vi "Query Slewrate Limits.vi"(7 "Channel (0: Channel A)":u16(ring) items=["Channel A", "Channel B"], 8 "error in (no error)":errorcluster, 11 "BH Druck PACE Series in":refnum<class "BH Druck PACE Series.lvclass">) -> (0 "error out":errorcluster, 1 "Lower Slew Rate Limit":dbl, 2 "Upper Slew Rate Limit":dbl, 3 "BH Druck PACE Series out":refnum<class "BH Druck PACE Series.lvclass">)   [LabVIEW 2022 SP3, in "BH Druck PACE Series.lvclass"]
uses:
  BH Druck PACE Series.lvclass
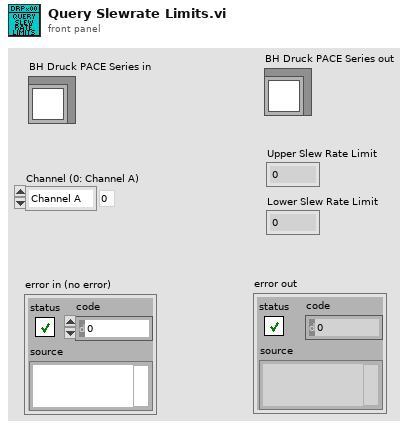
[diagram p1: front panel]
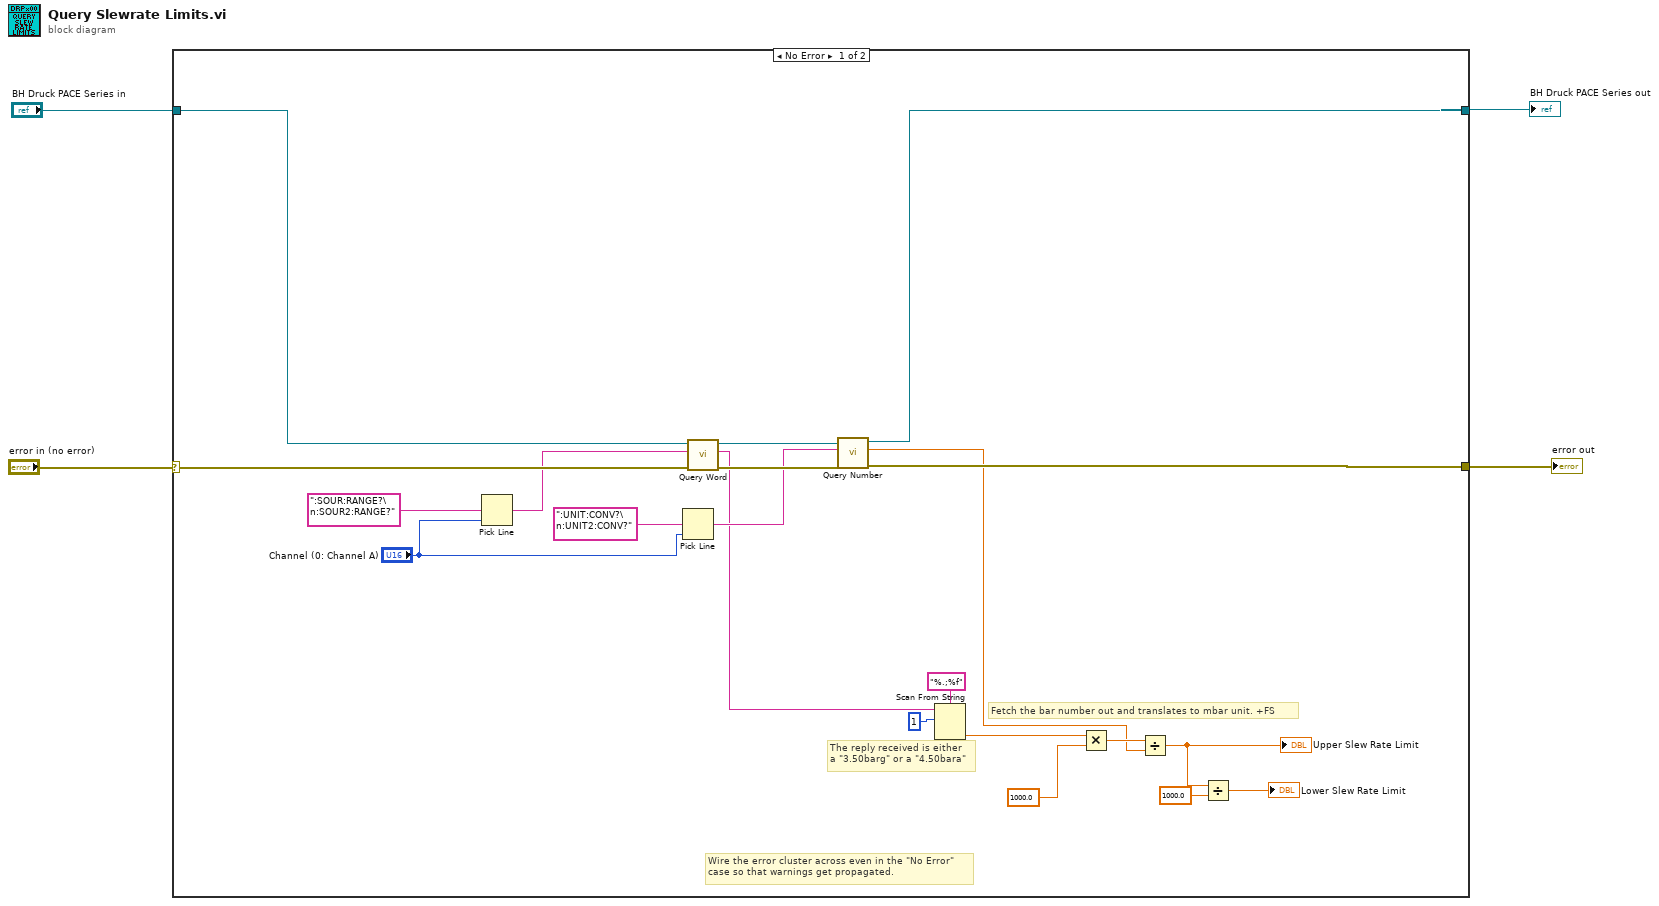
[diagram p0: block diagram]
diagram:
  n1 = case shown="No Error" "error in (no error)" {
    selector: "error in (no error)" -> [w22 w27]
    tunnel: [w20 w27] -> w3
    tunnel: [w16 w26] -> w1
    tunnel: "BH Druck PACE Series in" -> [w19 w26]
    frame No Error {
      # "Fetch the bar number out and translates to mbar unit. +FS"
      # "The reply received is either \na \"3.50barg\" or a \"4.50bara\""
      # "Wire the error cluster across even in the \"No Error\"\ncase so that warnings get propagated."
      n2 = Pick Line(multi-line string=":SOUR:RANGE?\n:SOUR2:RANGE?", line index="Channel (0: Channel A)") -> (output string=w15:string)  [unwired: 1 in]
      n3 = Pick Line(multi-line string=":UNIT:CONV?\n:UNIT2:CONV?", line index="Channel (0: Channel A)") -> (output string=w17:string)  [unwired: 1 in]
      n4 = call-dynamic "Query Word.vi"("error in (no error)"=w22, "Query String"=w15, "BH Druck PACE Series in"=w19) -> ("error out"=w21:errorcluster, "String Result"=w6:string, "BH Druck PACE Series out"=w18:refnum<class "BH Druck PACE Series.lvclass">)  [unwired: 6 in]
      n5 = call-dynamic "Query Number.vi"("error in (no error)"=w21, "Query String"=w17, "BH Druck PACE Series in"=w18) -> ("error out"=w20:errorcluster, "Numeric Result"=w5:dbl, "BH Druck PACE Series out"=w16:refnum<class "BH Druck PACE Series.lvclass">)  [unwired: 6 in]
      n6 = Scan From String(format string="%.;%f", input string=w6, initial scan location=u32 1) -> (output 1=w12:dbl)  [unwired: 2 in, 3 out]
      n7 = Multiply(x=w12, y=1000.0) -> (x*y=w10:dbl)
      n8 = Divide(x=w10, y=w5) -> (x/y=w9:dbl)
      "Upper Slew Rate Limit" <- w9
      n9 = Divide(x=w9, y=1000.0) -> (x/y=→"Lower Slew Rate Limit":dbl)
    }
    frame Error {
    }
  }
  "error out" <- w3
  "BH Druck PACE Series out" <- w1
